vi "Remote Video stream.vi"(1 "Quality":i32=750 min=0 max=1000, 2 "Camera":T1="Travcam") -> (0 "Error out":errorcluster)   [LabVIEW 2015]
uses:
  Camera enum/Camera enum.ctl
  Globals/CamServer global.vi
panel:
  # "PN 21/08/15"
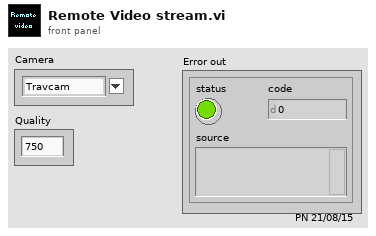
[diagram p1: front panel]
types:
  T1 = typedef "Camera enum.ctl" = string
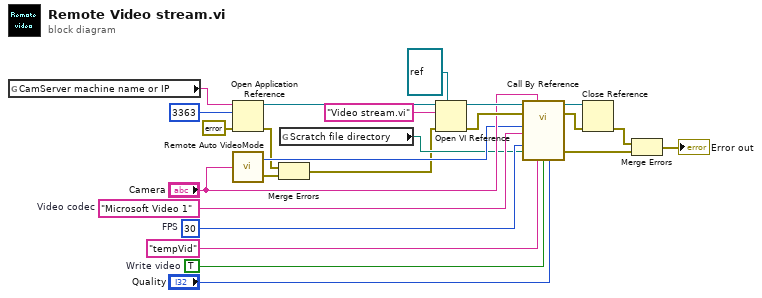
[diagram p0: block diagram]
diagram:
  w7 = "Microsoft Video 1"  # Video codec
  w8 = u32 30  # FPS
  w9 = TRUE  # Write video
  n1 = global read "CamServer global.vi" "CamServer machine name or IP"() -> (w6:string)
  n2 = Open Application Reference(8:errorcluster {"status"=FALSE, "code"=0, "source"=""} ("error in (no error)"), 10:u16 3363 ("port"), 11:w6) -> (0:w4:errorcluster, 3:w22:refnum<vi>)  [unwired: 1 in]
  n3 = call "Remote Auto VideoMode.vi"("Camera"="Camera") -> ("VideoMode"=w12:u32, "Error out"=w3:errorcluster)
  n4 = Merge Errors(w4, w3) -> (w2:errorcluster)
  n5 = global read "CamServer global.vi" "Scratch file directory"() -> (w5:path)
  n6 = Open VI Reference(type specifier VI Refnum (for type only)=refnum<vi> refnum, application reference (local)=w22, vi path="Video stream.vi" ("machine name"), error in (no error)=w2) -> (vi reference=w20:refnum<vi>, error out=w21:errorcluster)  [unwired: 2 in]
  n7 = call-by-ref "?"(reference=w20, error in=w21, "VideoMode"=w12, "Interface name"="Camera", "Video codec"=w7, "FPS"=w8, "Video directory path"=w5, "Video name"="tempVid" ("Image name"), "Write video"=w9, "Quality"="Quality") -> (reference out=w18:refnum<vi>, error out=w17:errorcluster, "Error Out"=w16:errorcluster)  [unwired: 7 in]
  n8 = Close Reference(reference=w18, error in (no error)=w17) -> (error out=w15:errorcluster)
  n9 = Merge Errors(w15, w16) -> (→"Error out":errorcluster)
